vi "CFG Build Cluster List.vi"(0 "Cluser Ref":refnum<vi>, 11 "Error in (no error)":errorcluster, 13 "Build Item Names (F)":bool) -> (4 "Item Refs":refnum<vi>[](array[refnum]), 6 "Item Names":string[](array[string]), 15 "error out":errorcluster)   [LabVIEW 2017]
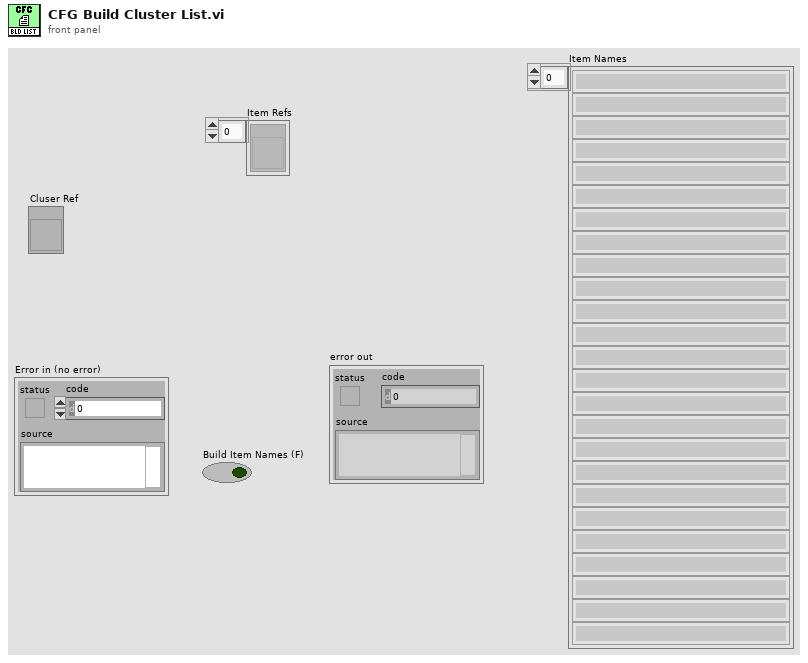
[diagram p1: front panel]
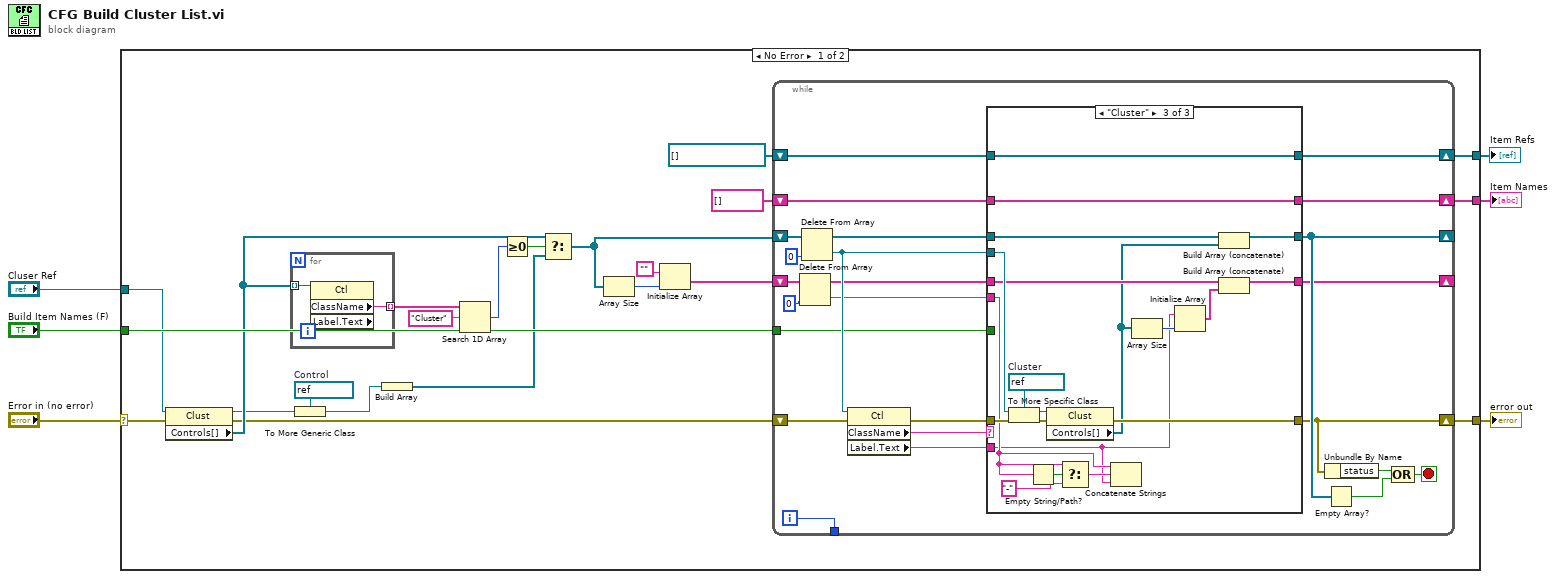
[diagram p0: block diagram]
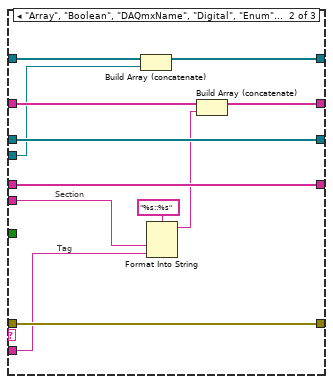
[diagram p3: hidden frame]
diagram:
  n1 = case shown="No Error" "Error in (no error)" {
    selector: "Error in (no error)" -> [w28 w92]
    tunnel: [w27 w92] -> w5
    tunnel: "Cluser Ref" -> [w11 _]
    tunnel: [w25 _] -> w4
    tunnel: [w24 _] -> w2
    tunnel: "Build Item Names (F)" -> [w23 _]
    frame No Error {
      w12 = refnum<vi> refnum  # Control
      n2 = property class="Clust"(reference=w11, error in=w28) -> (reference out=w10:refnum<vi>, error out=w8:errorcluster, "Controls[]"=w14:refnum<vi>[])
      n3 = for {
        tunnel: w14 -> [w30] mode=indexing
        tunnel: [w29] -> w18 mode=indexing
        n4 = property class="Ctl" props=["ClassName", "Label", "Text"](reference=w30) -> ("ClassName"=w29:string)  [unwired: 1 in, 3 out]
      }
      n5 = To More Generic Class(target class=w12, reference=w10) -> (generic class reference=w9:refnum<vi>)
      n6 = Build Array(w9) -> (w13:refnum<vi>[])
      n7 = Search 1D Array(1D array=w18, element="Cluster") -> (index of element=w16:i32)  [unwired: 1 in]
      n8 = Greater Or Equal To 0?(x=w16) -> (x >= 0?=w15:bool)
      n9 = Select(t=w14, s=w15, f=w13) -> (s? t:f=w7:refnum<vi>[])
      n10 = Array Size(array=w7) -> (size(s)=w22:i32)
      n11 = Initialize Array("", w22) -> (w21:string[])
      n12 = while {
        shift-right: [w47] -> w27
        shift-left: w8 -> [w52]
        shift-right: [w48] -> _
        shift-left: w7 -> [w53]
        shift-right: [w43] -> w25
        shift-left: string[] [] -> [w42]
        shift-right: [w41] -> w24
        shift-left: refnum<vi>[] [] -> [w40]
        tunnel: [w38] -> _
        tunnel: w23 -> [w37]
        shift-right: [w32] -> _
        shift-left: w21 -> [w34]
        i -> [w38]
        stop <- w44 stop-if-true
        n13 = Delete From Array(array=w34, index=0) -> (deleted portion=w31:string, array with subset deleted=w33:string[])  [unwired: 1 in]
        n14 = Delete From Array(array=w53, index=0) -> (deleted portion=w49:refnum<vi>, array with subset deleted=w35:refnum<vi>[])  [unwired: 1 in]
        n15 = property class="Ctl"(reference=w49, error in=w52) -> (error out=w50:errorcluster, "ClassName"=w54:string, "Label.Text"=w51:string)  [unwired: 1 out]
        n16 = case shown="\"Cluster\"" w54 {
          tunnel: w51 -> [_ w60 w72]
          tunnel: w35 -> [w58 w68 w91]
          tunnel: w50 -> [w59 w71 w90]
          tunnel: [w59 w71 w86] -> w47
          tunnel: [w58 w68 w84] -> w48
          tunnel: w49 -> [_ w65 w85]
          tunnel: [w56 w70 w83] -> w43
          tunnel: w42 -> [w56 w69 w83]
          tunnel: [w57 w67 w82] -> w41
          tunnel: w40 -> [w57 w66 w82]
          tunnel: w37 -> [_ _ _]
          tunnel: w33 -> [w55 w64 w81]
          tunnel: [w55 w64 w77] -> w32
          tunnel: w31 -> [_ w61 w73]
          frame Default {
          }
          frame "Array", "Boolean", "DAQmxName", "Digital", "Enum", "Path", "Slide", "String", "VISAResourceName" {
            # "Tag"
            # "Section"
            n17 = Build Array (concatenate)(w66, w65) -> (w67:refnum<vi>[])
            n18 = Format Into String(format string="%s::%s", w61, w60) -> (resulting string=w62:string)  [unwired: 2 in, 1 out]
            n19 = Build Array (concatenate)(w69, w62) -> (w70:string[])
          }
          frame "Cluster" {
            w87 = refnum<vi> refnum  # Cluster
            n20 = To More Specific Class(target class=w87, reference=w85, error in=w90) -> (specific class reference=w88:refnum<vi>, error out=w89:errorcluster)
            n21 = Empty String/Path?(string/path=w73) -> (empty?=w76:bool)
            n22 = property class="Clust"(reference=w88, error in=w89) -> (error out=w86:errorcluster, "Controls[]"=w79:refnum<vi>[])  [unwired: 1 out]
            n23 = Select(t=w73, s=w76, f="-") -> (s? t:f=w74:string)
            n24 = Concatenate Strings(w73, w74, w72) -> ()  [unwired: 1 out]
            n25 = Array Size(array=w79) -> (size(s)=w80:i32)
            n26 = Initialize Array(w72, w80) -> (w78:string[])
            n27 = Build Array (concatenate)(w91, w79) -> (w84:refnum<vi>[])
            n28 = Build Array (concatenate)(w81, w78) -> (w77:string[])
          }
        }
        n29 = Unbundle By Name(w47) -> ("status"=w46:bool)
        n30 = Empty Array?(array=w48) -> (empty?=w45:bool)
        n31 = Compound Arithmetic op=OR(w46, w45) -> (w44:bool)
      }
    }
    frame Error {
    }
  }
  "error out" <- w5
  "Item Names" <- w4
  "Item Refs" <- w2
